vi "SubVI FM Demodulation Differentiate - Continuous.vi"(3 "输入信号":waveform(dbl)) -> (1 "dx/dt":waveform(dbl))   [LabVIEW 2015]
uses:
  <vilib>/ptbypt/NI_PtbyPt.lvlib
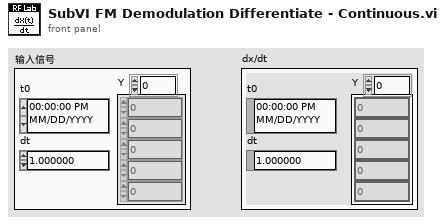
[diagram p1: front panel]
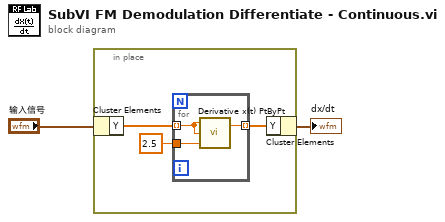
[diagram p0: block diagram]
diagram:
  n1 = in-place {
    n2 = in-place-cluster #1("输入信号") -> ("Y"=w4:dbl[])
    n3 = for {
      tunnel: w4 -> [w7] mode=indexing
      tunnel: [w8] -> w3 mode=indexing
      tunnel: 2.5 ("dx/dt") -> [w6]
      n4 = call <vilib>:"Derivative x(t) PtByPt.vi"("dt"=w6, "initial condition"=w7, "x"=w7) -> ("dx/dt"=w8:dbl)  [unwired: 1 in, 1 out]
    }
    n5 = in-place-cluster #1("Y"=w3) -> (→"dx/dt":waveform(dbl))
  }
